vi "Function.vi"(8 "error in (no error)":errorcluster, 10 "Value":ext, 11 "Two Terminal in":refnum<class "Decrement_EXT.lvclass">) -> (0 "error out":errorcluster, 2 "Result":ext, 3 "Two Terminal out":refnum<class "Decrement_EXT.lvclass">)   [LabVIEW 2021, in "Decrement_EXT.lvclass"]
uses:
  Decrement_EXT.lvclass
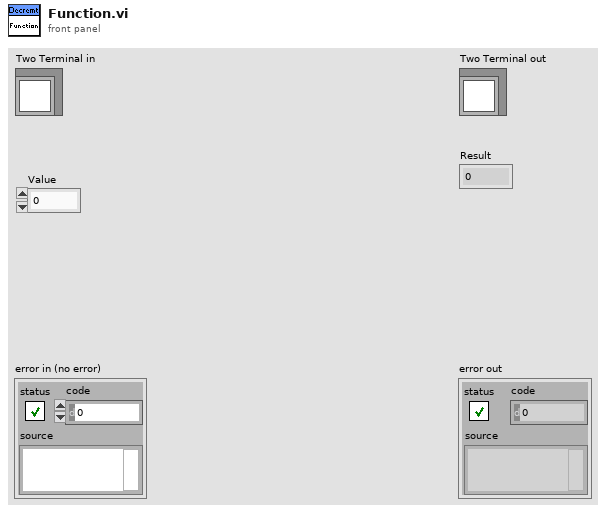
[diagram p1: front panel]
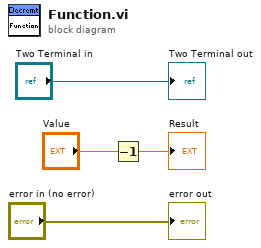
[diagram p0: block diagram]
diagram:
  n1 = Decrement(x="Value") -> (x-1=→"Result":ext)
  "error out" <- "error in (no error)"
  "Two Terminal out" <- "Two Terminal in"
